vi "AGCxxx Command restart.vi"(7 "error in (no error)":errorcluster, 10 "AGCxxx VISA Cluster":T1={"VISA resource name"="", "VISA Timeout Value (1000 ms)"=1000, "Lock Timeout (1000 ms)"=1000, "MAX Channel (6)"=6}) -> (0 "error out":errorcluster, 1 "AGC Errno":i32, 3 "dup AGCxxx VISA Cluster":T1={"VISA resource name"="", "VISA Timeout Value (1000 ms)"=1000, "Lock Timeout (1000 ms)"=1000, "MAX Channel (6)"=6})   [LabVIEW 2014, in "AGCxxx - Driver.lvlib"]
doc: "This causes the AGC to restart operation as if the electrical sypply had benn switched off, then on again.\n! THE AGC NEEDS 12 SECONDS TO RESTART !\n\nCopyright (C) \nGesellschaft f. Schwerionenforschung, GSI\nPlanckstr. 1\n64291 Darmstadt\nGermany\n\nContact: http://www-wnt.gsi.de/labview\n H.Brand@gsi.de\n\nThis program is free software; you can redistribute it and/or\nmodify it under the terms of the GNU General Public License\nas published by the Free Software Foundation; either version 2\nof the License, or (at your option) any later version.\n\nThis program is distributed in the hope that it will be useful,\nbut WITHOUT ANY WARRANTY; without even the implied warranty of\nMERCHANTABILITY or FITNESS FOR A PARTICULAR PURPOSE. See the\nGNU General Public License for more details (http://www.gnu.org)."
uses:
  AGCxxx - Driver.lvlib
  AGCxxx VISA Control.ctl
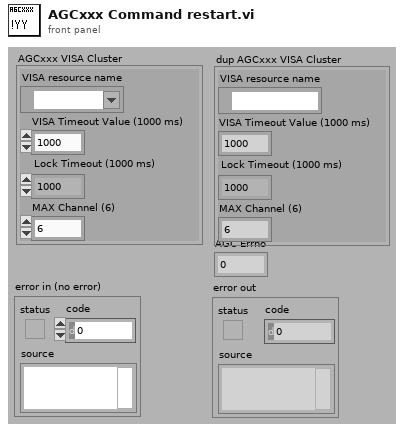
[diagram p1: front panel]
types:
  T1 = typedef "AGCxxx - Driver.lvlib/AGCxxx VISA Control.ctl" = cluster{"VISA resource name":refnum<visa-resource-name>, "VISA Timeout Value (1000 ms)":u32, "Lock Timeout (1000 ms)":u32, "MAX Channel (6)":i32}
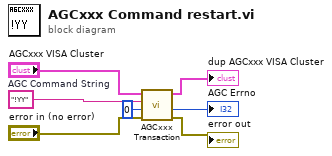
[diagram p0: block diagram]
diagram:
  w2 = "!YY"  # AGC Command String
  n1 = call "AGCxxx Transaction.vi"("error in (no error)"="error in (no error)", "Bytes to read (100)"=u32 0, "AGC Command String"=w2, "AGCxxx VISA Cluster"="AGCxxx VISA Cluster") -> ("error out"=→"error out":errorcluster, "AGC Errno"=→"AGC Errno":i32, "dup AGCxxx VISA Cluster"=→"dup AGCxxx VISA Cluster":T1)  [unwired: 3 in, 1 out]
